vi "Load Input File.vi"(8 "error in (no error)":errorcluster, 10 "Path":path, 11 "LBCB Filter":T3) -> (0 "error out":errorcluster, 2 "Load Steps":T1[](array[typedef]))   [LabVIEW 2013]
uses:
  Data Access Objects/Metadata/LBCB Number.ctl
  MixedMode/Load Step.ctl
  MixedMode/Messages/Target.ctl
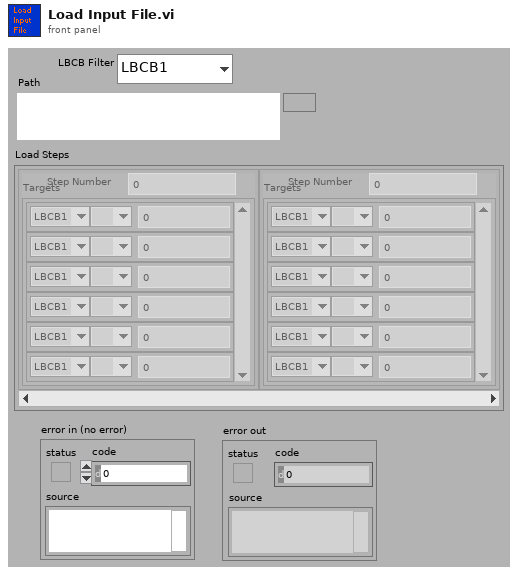
[diagram p1: front panel]
types:
  T1 = typedef "Load Step.ctl" = cluster{"Step Number":u32, "Targets":T2[]}
  T2 = typedef "Target.ctl" = cluster{"LBCB Number":T3, "DOF Vectors":enum16{" ", "Dx", "Dy", "Dz", "Rx", "Ry", "Rz", "Fx", "Fy", "Fz", "Mx", "My", "Mz"}, "Amount":dbl}
  T3 = typedef "LBCB Number.ctl" = enum16{"LBCB1", "LBCB2"}
  T4 = enum16{" ", "Dx", "Dy", "Dz", "Rx", "Ry", "Rz", "Fx", "Fy", "Fz", "Mx", "My", "Mz"}[]
  T5 = enum16{"open", "replace", "create", "open or create", "replace or create", "replace or create with confirmation"}
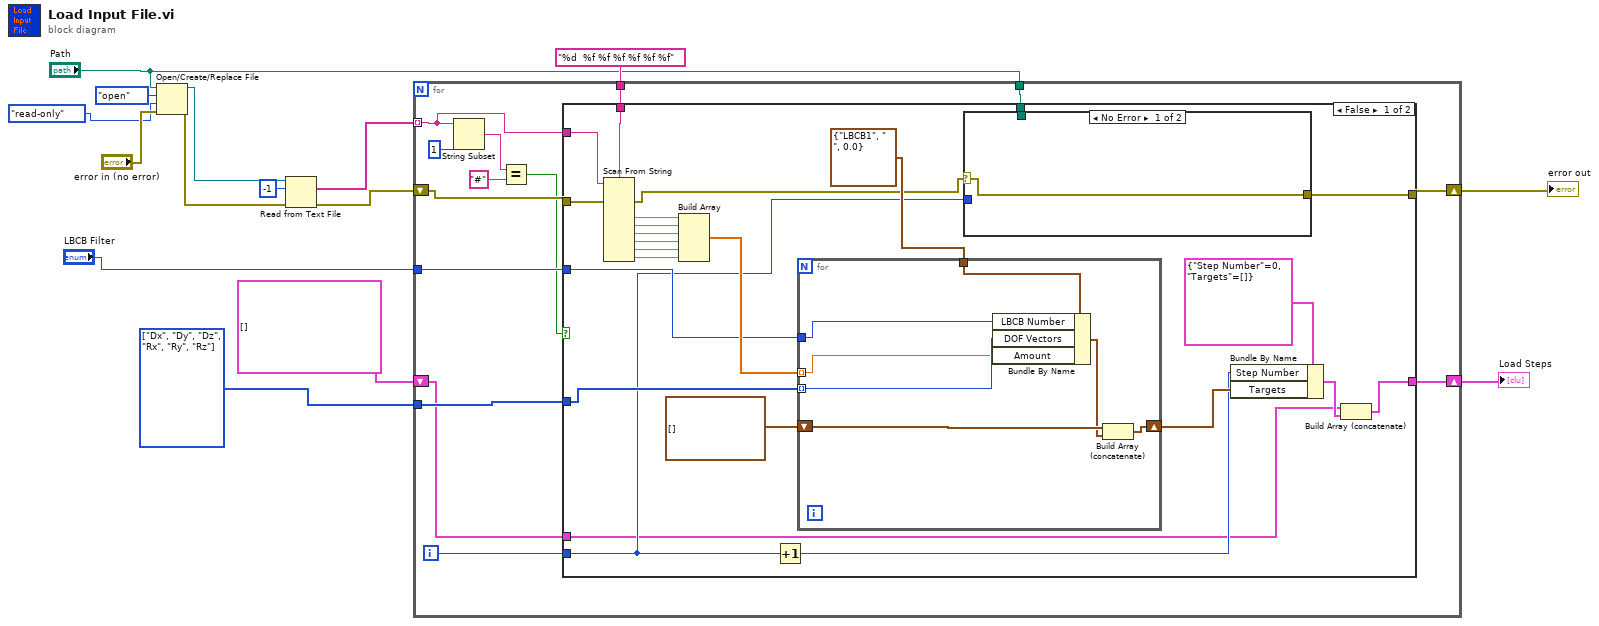
[diagram p0: block diagram]
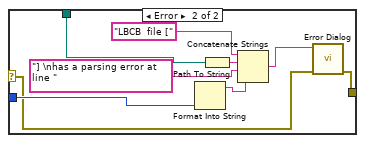
[diagram p2: hidden frame]
diagram:
  w10 = T4 [enum."Dx", enum."Dy", enum."Dz", enum."Rx", enum."Ry", enum."Rz"] items=[" ", "Dx", "Dy", "Dz", "Rx", "Ry", "Rz", "Fx", "Fy", "Fz", "Mx", "My", "Mz"]
  n1 = Open/Create/Replace File(file path (use dialog)="Path", error in="error in (no error)", operation (0:open)=T5."open", access (0:read/write)=enum16{"read/write", "read-only", "write-only"}."read-only") -> (refnum out=w14:refnum<file>, error out=w6:errorcluster)  [unwired: 3 out]
  n2 = Read from Text File(file (use dialog)=w14, count=-1, error in=w6) -> (text=w12:string[], error out=w5:errorcluster)  [unwired: 3 out]
  n3 = for {
    tunnel: w12 -> [w20] mode=indexing
    tunnel: "LBCB Filter" -> [w29]
    tunnel: w10 -> [w28]
    tunnel: "%d  %f %f %f %f %f %f" ("format string") -> [w26]
    shift-right: [w24] -> w4
    shift-left: w5 -> [w25]
    tunnel: "Path" -> [w22]
    shift-right: [w27] -> w9
    shift-left: cluster{"Step Number":u32, "Targets":T2[]}[] [] -> [w16]
    i -> [w23]
    n4 = String Subset(string=w20, length (rest)=1 ("length (rest)")) -> (substring=w19:string)  [unwired: 1 in]
    n5 = Equal?(x=w19, y="#") -> (x = y?=w17:bool)
    n6 = case shown="False" w17 {
      tunnel: w20 -> [w53 _]
      tunnel: w29 -> [w44 _]
      tunnel: w28 -> [w43 _]
      tunnel: [w31 w71] -> w27
      tunnel: w26 -> [w39 _]
      tunnel: w25 -> [w38 w72]
      tunnel: [w34 w72] -> w24
      tunnel: w23 -> [w36 _]
      tunnel: w22 -> [w33 _]
      tunnel: w16 -> [w30 w71]
      frame False {
        n7 = Scan From String(format string=w39, input string=w53, error in=w38) -> (error out=w35:errorcluster, output 2=w52:dbl, output 3=w51:dbl, output 4=w50:dbl, output 5=w49:dbl, output 6=w48:dbl, output 7=w47:dbl)  [unwired: 1 in, 10 out]
        n8 = Build Array(w52, w51, w50, w49, w48, w47) -> (w46:dbl[])
        n9 = Increment(x=w36) -> (x+1=w37:i32)
        n10 = for {
          tunnel: w46 -> [w67] mode=indexing
          tunnel: T2 {"LBCB Number"=enum."LBCB1", "DOF Vectors"=enum." ", "Amount"=0.0} ("Target") -> [w70]
          tunnel: w44 -> [w69]
          tunnel: w43 -> [w68] mode=indexing
          shift-right: [w66] -> w40
          shift-left: T2[] [] -> [w65]
          n11 = Bundle By Name(cluster=w70, "LBCB Number"=w69, "DOF Vectors"=w68, "Amount"=w67) -> (w64:T2)
          n12 = Build Array (concatenate)(w65, w64) -> (w66:T2[])
        }
        n13 = case shown="No Error" w35 {
          selector: w35 -> [w54 w55]
          tunnel: w36 -> [_ w59]
          tunnel: [w54 w57] -> w34
          tunnel: w33 -> [_ w56]
          frame No Error {
          }
          frame Error {
            n14 = Format Into String(w59) -> (resulting string=w58:string)  [unwired: 3 in, 1 out]
            n15 = Path To String(path=w56) -> (string=w60:string)
            n16 = Concatenate Strings("LBCB  file [" ("string"), w60, "] \nhas a parsing error at line " ("string"), w58) -> (w61:string)
            n17 = call "Error Dialog.vi"("error in (no error)"=w55, "Message"=w61) -> ("error out"=w57:errorcluster)  [unwired: 9 out]
          }
        }
        n18 = Bundle By Name(cluster=cluster{"Step Number":u32, "Targets":T2[]} {"Step Number"=0, "Targets"=[]} ("Load Step"), "Step Number"=w37, "Targets"=w40) -> (w32:cluster{"Step Number":u32, "Targets":T2[]})
        n19 = Build Array (concatenate)(w30, w32) -> (w31:cluster{"Step Number":u32, "Targets":T2[]}[])
      }
      frame True {
      }
    }
  }
  "Load Steps" <- w9
  "error out" <- w4
